vi "EDS test 01_with motor.vi"() -> ()   [LabVIEW 2020]
uses:
  <vilib>/Instr/_visa.llb/VISA Configure Serial Port (Instr).vi
panel:
  out "concatenated string":string
  out "US 2":string
  out "US 1":string
  out "read buffer":string
  in  "stop":bool
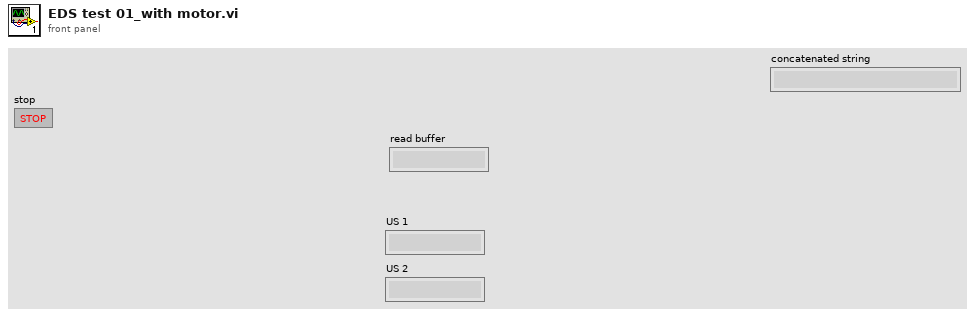
[diagram p1: front panel]
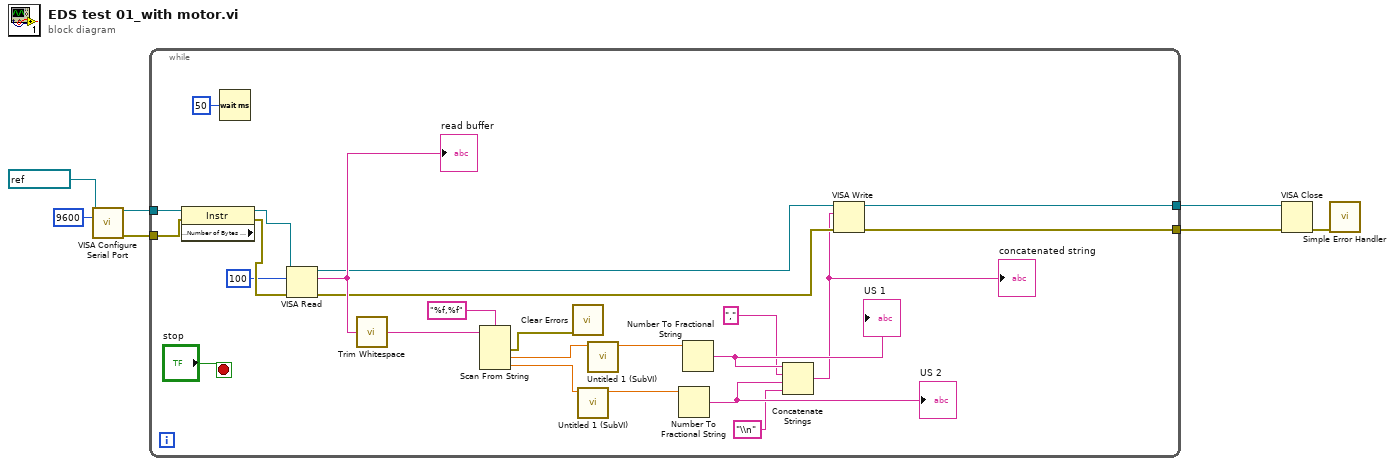
[diagram p0: block diagram]
diagram:
  n1 = call-poly "VISA Configure Serial Port"("VISA resource name"=refnum<visa-resource-name> "COM3", "baud rate (9600)"=u32 9600) -> ("VISA resource name out"=w5:refnum<visa-resource-name>, "error out"=w4:errorcluster)  [unwired: 12 in]
  n2 = while {
    tunnel: w5 -> [w31]
    tunnel: w4 -> [w30]
    tunnel: [w13] -> w2
    tunnel: [w12] -> w1
    stop <- "stop" stop-if-true
    n3 = property class="Instr" props=["Serial Settings:Number of Bytes at Serial Port"](reference=w31, error in=w30) -> (reference out=w26:refnum<visa-resource-name>, error out=w27:errorcluster)  [unwired: 1 out]
    n4 = Wait (ms)(milliseconds to wait=u32 50) -> ()  [unwired: 1 out]
    n5 = VISA Read(VISA resource name=w26, byte count=u32 100, error in (no error)=w27) -> (VISA resource name out=w15:refnum<visa-resource-name>, read buffer=w25:string, error out=w14:errorcluster)  [unwired: 1 out]
    "read buffer" <- w25
    n6 = call <vilib>:"Trim Whitespace.vi"("string"=w25) -> ("trimmed string"=w24:string)  [unwired: 1 in]
    n7 = Scan From String(format string="%f,%f", input string=w24) -> (error out=w22:errorcluster, output 1=w20:dbl, output 2=w19:dbl)  [unwired: 4 in, 2 out]
    n8 = call <vilib>:"Clear Errors.vi"("error in (no error)"=w22) -> ()  [unwired: 5 in, 2 out]
    n9 = call "Untitled 1 (SubVI).vi"("Ultrasonic 01"=w19) -> ("Numeric"=w17:dbl)  [unwired: 10 in]
    n10 = call "Untitled 1 (SubVI).vi"("Ultrasonic 01"=w20) -> ("Numeric"=w18:dbl)  [unwired: 10 in]
    n11 = Number To Fractional String(number=w17) -> (F-format string=w10:string)  [unwired: 3 in]
    "US 2" <- w10
    n12 = Number To Fractional String(number=w18) -> (F-format string=w16:string)  [unwired: 3 in]
    "US 1" <- w16
    n13 = Concatenate Strings(w16, ",", w10, "\\n") -> (w11:string)
    "concatenated string" <- w11
    n14 = VISA Write(VISA resource name=w15, write buffer=w11, error in (no error)=w14) -> (VISA resource name out=w13:refnum<visa-resource-name>, error out=w12:errorcluster)  [unwired: 1 out]
  }
  n15 = VISA Close(VISA resource name=w2, error in (no error)=w1) -> (error out=w3:errorcluster)
  n16 = call <vilib>:"Simple Error Handler.vi"("error in (no error)"=w3) -> ()  [unwired: 4 in, 5 out]
